vi "milliGAT Configure and Run.vi"() -> ()   [LabVIEW 2015]
uses:
  Global FIA milliGAT.lvlib
  Public/Utility/Pump Direction.ctl
  Public/Utility/Pump Address.ctl
panel:
  in  "Flow Patameters":T1={"Peak Flow (uL/s)"=100.0, "Starting Flow (uL/s)"=0.1, "Acceleration (uL/s^2)"=500.0, "Deceleration (uL/s^2)"=500.0}
  in  "Action":T2
  in  "Pump ID (0:A)":T3
  in  "Serial Configuration":cluster{"Baud Rate":u32}={"Baud Rate"=9600} {"Baud Rate" items=["300"=300, "600"=600, "1200"=1200, "2400"=2400, "4800"=4800, "9600"=9600, "19200"=19200]}
  out "Microliters":dbl
  in  "Volume (0 uL)":dbl
  out "error out":errorcluster
  in  "VISA resource name":refnum<visa-resource-name>="COM1"
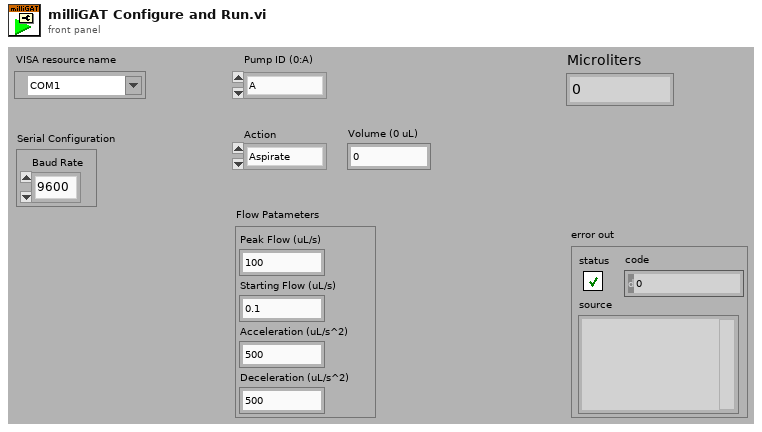
[diagram p1: front panel]
types:
  T1 = cluster{"Peak Flow (uL/s)":dbl, "Starting Flow (uL/s)":dbl, "Acceleration (uL/s^2)":dbl, "Deceleration (uL/s^2)":dbl}
  T2 = typedef "Global FIA milliGAT.lvlib/Pump Direction.ctl" = enum16{"Aspirate", "Dispense"}
  T3 = typedef "Global FIA milliGAT.lvlib/Pump Address.ctl" = enum16{"A", "B", "C", "D", "E", "F", "G", "H", "I", "J", "K", "L", "M", "N", "O", "P", "Q", "R", "S", "T", "U", "V", "W", "X", "Y", "Z", "a", "b", "c", "d", "e", "f", "g", "h", "i", "j", "k", "l", "m", "n", "o", "p", "q", "r", "s", "t", "u", "v", "w", "x", "y", "z", "0", "1", "2", "3", "4", "5", "6", "7", "8", "9"}
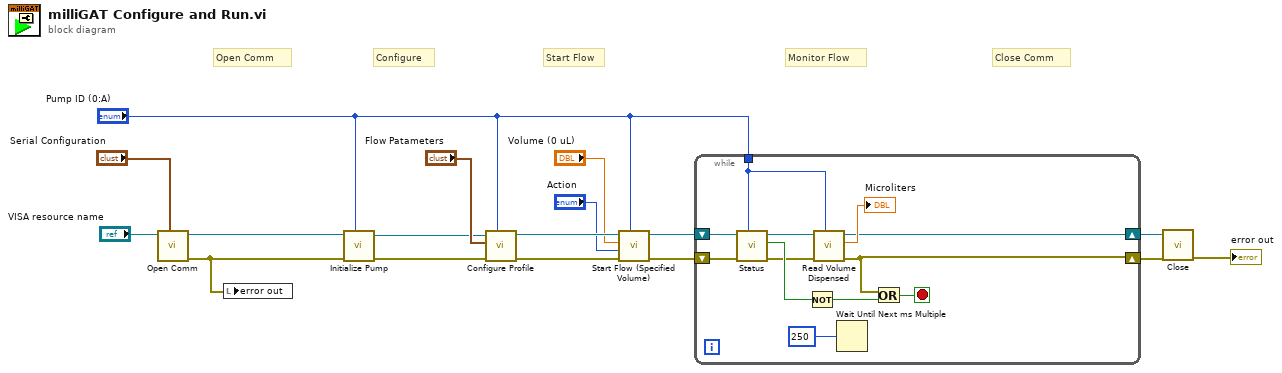
[diagram p0: block diagram]
diagram:
  # "Start Flow"
  # "Open Comm"
  # "Configure"
  # "Monitor Flow"
  # "Close Comm"
  n1 = call "Open Comm.vi"("Serial Configuration"="Serial Configuration", "VISA resource in"="VISA resource name") -> ("error out"=w1:errorcluster, "VISA resource out"=w10:refnum<visa-resource-name>)  [unwired: 8 in]
  n2 = local write "error out"(w1) -> ()
  n3 = call "Initialize Pump.vi"("Pump ID (0:A)"="Pump ID (0:A)", "error in (no error)"=w1, "VISA resource in"=w10) -> ("error out"=w5:errorcluster, "VISA resource out"=w6:refnum<visa-resource-name>)  [unwired: 7 in]
  n4 = call "Configure Profile.vi"("Pump ID (0:A)"="Pump ID (0:A)", "error in (no error)"=w5, "Flow Parameters"="Flow Patameters", "VISA resource in"=w6) -> ("error out"=w15:errorcluster, "VISA resource out"=w17:refnum<visa-resource-name>)  [unwired: 6 in]
  n5 = call "Start Flow (Specified Volume).vi"("Pump ID (0:A)"="Pump ID (0:A)", "error in (no error)"=w15, "Direction (0: Aspirate)"="Action", "Volume (0 uL)"="Volume (0 uL)", "VISA resource in"=w17) -> ("error out"=w7:errorcluster, "VISA resource out"=w14:refnum<visa-resource-name>)  [unwired: 5 in]
  n6 = while {
    shift-right: [w19] -> w2
    shift-left: w14 -> [w26]
    tunnel: "Pump ID (0:A)" -> [w20]
    shift-right: [w18] -> w3
    shift-left: w7 -> [w27]
    stop <- w22 stop-if-true
    n7 = call "Status.vi"("Pump ID (0:A)"=w20, "error in (no error)"=w27, "VISA resource in"=w26) -> ("error out"=w24:errorcluster, "moving"=w29:bool, "VISA resource out"=w25:refnum<visa-resource-name>)  [unwired: 6 in]
    n8 = Not(x=w29) -> (.not. x?=w23:bool)
    n9 = call "Read Volume Dispensed.vi"("Pump ID (0:A)"=w20, "error in (no error)"=w24, "VISA resource in"=w25) -> ("error out"=w18:errorcluster, "microliters"=→"Microliters":dbl, "VISA resource out"=w19:refnum<visa-resource-name>)  [unwired: 6 in]
    n10 = Wait Until Next ms Multiple(millisecond multiple=u32 250) -> ()  [unwired: 1 out]
    n11 = Or(x=w18, y=w23) -> (x .or. y?=w22:bool)
  }
  n12 = call "Close.vi"("error in (no error)"=w3, "VISA resource in"=w2) -> ("error out"=→"error out":errorcluster)  [unwired: 9 in]
